vi "4Pi Obj Lock - 1 Values Organize Plot Data.vi"(0 "Target 01":dbl, 2 "Value Limit":dbl, 9 "Current 01":dbl) -> (8 "Plot Data":T1)   [LabVIEW 2021]
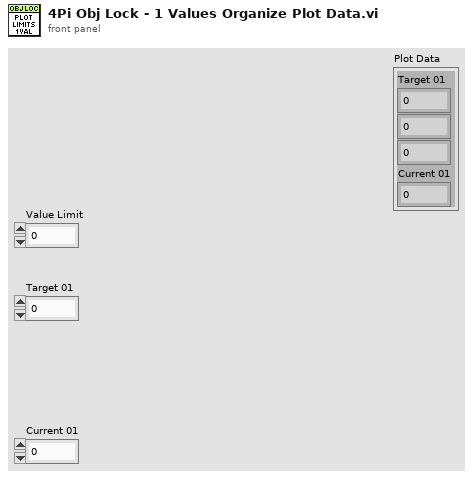
[diagram p1: front panel]
types:
  T1 = cluster{"Target 01":dbl, dbl, dbl, "Current 01":dbl}
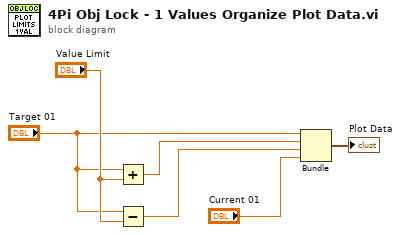
[diagram p0: block diagram]
diagram:
  n1 = Add(x="Target 01", y="Value Limit") -> (x+y=w4:dbl)
  n2 = Subtract(x="Target 01", y="Value Limit") -> (x-y=w3:dbl)
  n3 = Bundle("Target 01"="Target 01", w4, w3, "Current 01"="Current 01") -> (→"Plot Data":T1)  [unwired: 1 in]
